vi "DAQ_Init.vi"(0 "object in":refnum<class "DAQ.lvclass">, 2 "ConfigNI":T1 {"Sample Mode" items=["Finite Samples"=10178, "Continuous Samples"=10123, "Hardware Timed Single Point"=12522]; "Input Terminal Configuration" items=["Default"=-1, "RSE"=10083, "NRSE"=10078, "Differential"=10106, "Pseudodifferential"=12529]}, 5 "error in (no error)":errorcluster) -> (14 "object out":refnum<class "DAQ.lvclass">, 19 "error out":errorcluster)   [LabVIEW 2021, in "DAQ.lvclass"]
uses:
  DAQ.lvclass
  ConfigNI.ctl
  DAQ.lvclass/DAQ.ctl
  <vilib>/DAQmx/create/channels.llb/DAQmx Create Channel (AI-Voltage-Basic).vi
  <vilib>/DAQmx/configure/timing.llb/DAQmx Timing (Sample Clock).vi
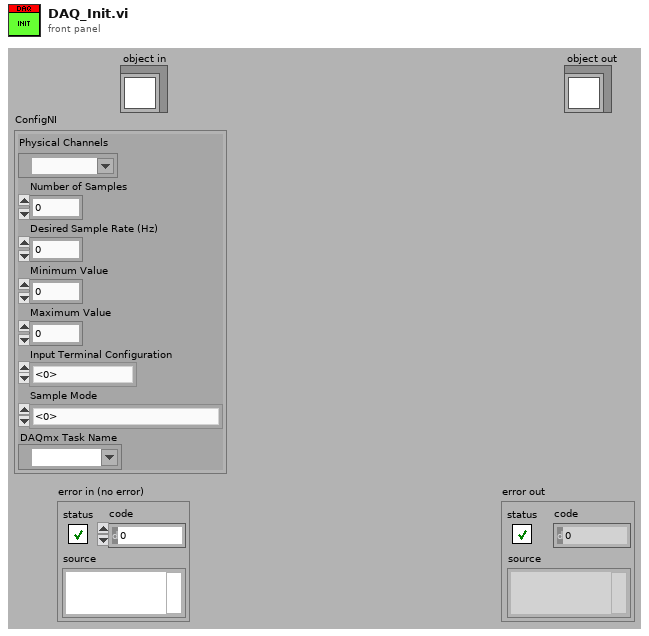
[diagram p1: front panel]
types:
  T1 = typedef "ConfigNI.ctl" = cluster{"Physical Channels":tag, "Number of Samples":i32, "Desired Sample Rate (Hz)":dbl, "Minimum Value":dbl, "Maximum Value":dbl, "Input Terminal Configuration":i32, "Sample Mode":i32, "DAQmx Task Name":refnum<k21>}
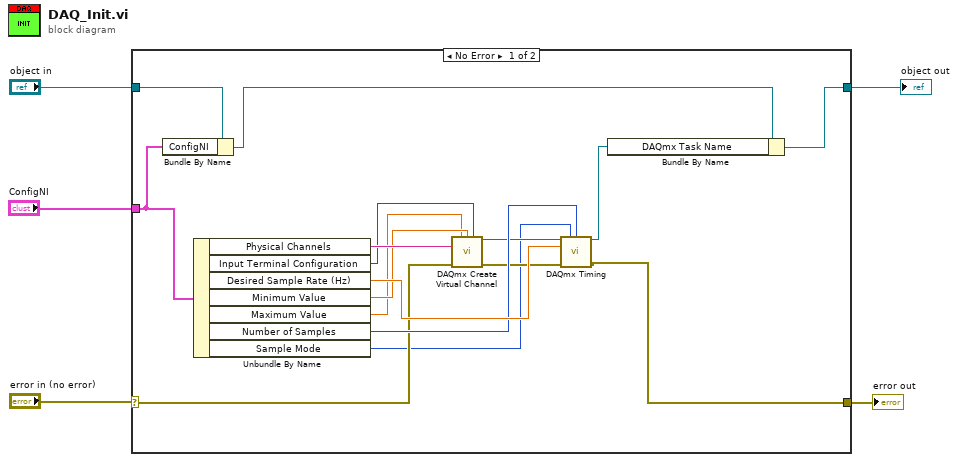
[diagram p0: block diagram]
diagram:
  n1 = case shown="No Error" "error in (no error)" {
    selector: "error in (no error)" -> [w14 w22]
    tunnel: "object in" -> [w21 w23]
    tunnel: [w10 w23] -> w4
    tunnel: [w13 w22] -> w2
    tunnel: "ConfigNI" -> [w20 _]
    frame No Error {
      n2 = Bundle By Name(cluster=w21, "ConfigNI"=w20) -> (w11:refnum<class "DAQ.lvclass">)
      n3 = Unbundle By Name(w20) -> ("Physical Channels"=w17:tag, "Input Terminal Configuration"=w9:i32, "Desired Sample Rate (Hz)"=w19:dbl, "Minimum Value"=w7:dbl, "Maximum Value"=w6:dbl, "Number of Samples"=w18:i32, "Sample Mode"=w8:i32)
      n4 = call-poly <vilib>:"DAQmx Create Virtual Channel.vi"("maximum value"=w6, "minimum value"=w7, "input terminal configuration"=w9, "physical channels"=w17, "error in"=w14) -> ("task out"=w16:refnum<k21>, "error out"=w15:errorcluster)  [unwired: 9 in]
      n5 = call-poly <vilib>:"DAQmx Timing.vi"("task/channels in"=w16, "sample mode"=w8, "samples per channel"=w18, "rate"=w19, "error in"=w15) -> ("task out"=w12:refnum<k21>, "error out"=w13:errorcluster)  [unwired: 9 in]
      n6 = Bundle By Name(cluster=w11, "DAQmx Task Name"=w12) -> (w10:refnum<class "DAQ.lvclass">)
    }
    frame Error {
    }
  }
  "object out" <- w4
  "error out" <- w2
